vi "STS_Add_PCU_CalData.vi"(8 "错误输入（无错误）":errorcluster, 10 "errorArray":sgl[][][](array[numeric]), 11 "STSProcess.PDLSTS":refnum<k24>) -> (0 "错误输出":errorcluster, 3 "PDLSTS out":refnum<k24>)   [LabVIEW 2017]
uses:
  D:/test/PDLSTS/LV_PDL LvVer17.0/LV_PDL_x86/DLL/STSProcess.dll
  DLL/STSProcess.dll
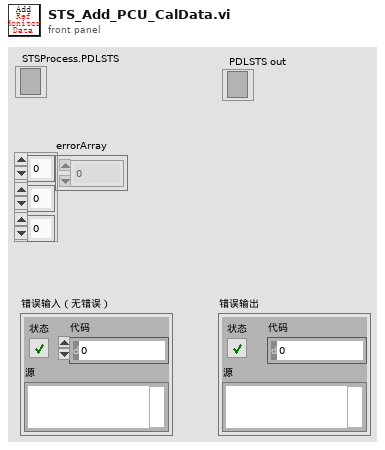
[diagram p1: front panel]
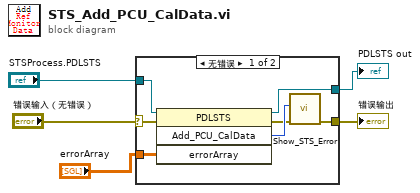
[diagram p0: block diagram]
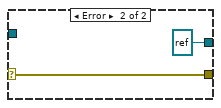
[diagram p2: hidden frame]
diagram:
  n1 = case shown="无错误" "错误输入（无错误）" {
    selector: "错误输入（无错误）" -> [w11 w14]
    tunnel: [w7 w14] -> w5
    tunnel: "STSProcess.PDLSTS" -> [w12 _]
    tunnel: [w10 refnum<k24> refnum ("STSProcess.PDLSTS")] -> w2
    tunnel: "errorArray" -> [w6 _]
    frame No Error {
      n2 = invoke on="调用节点" class="PDLSTS" method="Add_PCU_CalData"(reference=w12, error in=w11, "errorArray"=w6) -> (reference out=w10:refnum<k24>, error out=w8:errorcluster, "Add_PCU_CalData"=w9:i32)  [unwired: 1 in, 1 out]
      n3 = call "Show_STS_Error.vi"("error in (no error)"=w8, "Error"=w9) -> ("error out"=w7:errorcluster)  [unwired: 9 in]
    }
    frame Error {
    }
  }
  "错误输出" <- w5
  "PDLSTS out" <- w2
